vi "DatabaseHand_Element_Set(double).vi"(1 "precision":i8=6, 4 "enqueue? (F)":bool, 5 "group":string, 6 "permissions":string="RW", 7 "name":string, 8 "error in (no error)":errorcluster, 9 "unit":string, 10 "value":dbl format="%.2f", 11 "Database RefNum in":T1) -> (0 "error out":errorcluster, 3 "Database RefNum out":T1)   [LabVIEW 2016]
doc: "This VI finds the RefNum of an existing object with the input Name or creates a new object if the Name is not found or Name is unwired or an empty string.\nCopyright 2001 VI Engineering, Inc."
uses:
  DatabaseHand_RefNum.ctl
  DatabaseHand_Function.ctl
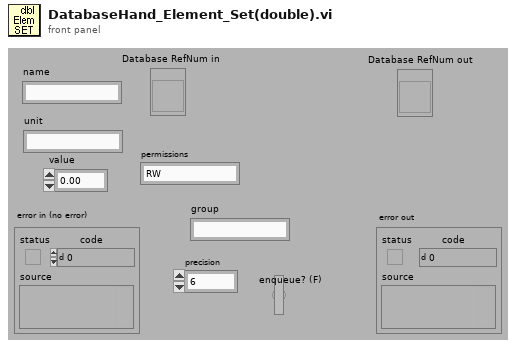
[diagram p1: front panel]
types:
  T1 = typedef "DatabaseHand_RefNum.ctl" = refnum<vi>
  T2 = typedef "DatabaseHand_Function.ctl" = enum16{"Reset", "Register", "Get Data", "Set Data", "Unregister", "Test", "Get Objects", "Delete Data"}
  T3 = typedef "DatabaseHand_Element.ctl" = cluster{"name":string, "Database":T4[]}
  T4 = typedef "DatabaseHan_DatabaseElement.ctl" = cluster{"name":string, "value":string, "type":string, "unit":string, "permissions":string, "enqueued":bool, "group":string}
  T5 = typedef "Database_Refnum.ctl" = refnum<vi>
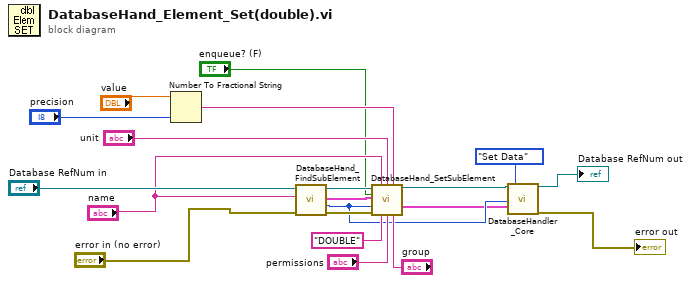
[diagram p0: block diagram]
diagram:
  n1 = Number To Fractional String(number="value", precision (6)="precision") -> (F-format string=w7:string)  [unwired: 2 out]
  n2 = call "DatabaseHand_FindSubElement.vi"("error in (no error)"="error in (no error)", "name"="name", "Database RefNum in"="Database RefNum in") -> ("error out"=w15:errorcluster, "index"=w4:i32, "Database"=w13:T3, "Database RefNum out"=w14:T1)  [unwired: 5 out]
  n3 = call "DatabaseHand_SetSubElement.vi"("Database RefNum in"=w14, "name"="name", "unit"="unit", "value"=w7, "enqueue? (F)"="enqueue? (F)", "Object Data In"=w13, "Index"=w4, "error in (no error)"=w15, "type"="DOUBLE", "permissions"="permissions", "group"="group") -> ("Database RefNum out"=w8:T1, "SubEle Out"=w3:T4)  [unwired: 3 out]
  n4 = call "DatabaseHandler_Core.vi"("Object Refnum In"=w8, "subele index"=w4, "SubEle In"=w3, "Function (Get Data)"=DatabaseHand_Function."Set Data") -> ("Object Refnum out"=→"Database RefNum out":T5, "error out"=→"error out":errorcluster)  [unwired: 3 in, 11 out]
